vi "Exit CMD.vi"(11 "Close Panel on Exit?":bool) -> (3 "Exit CMD":string)   [LabVIEW 2017]
doc: "函数名称： \n函数功能：JKI状态机 退出命令 （退出前输出输出数据） \n入口参数：\n出口参数：\n创建时间：2018-8-14 编辑者 ：翁赟\n---------------------------------------------------------------------\n修改时间：\n修改备注： 注意状态机里 命令是否符合"
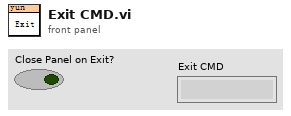
[diagram p1: front panel]
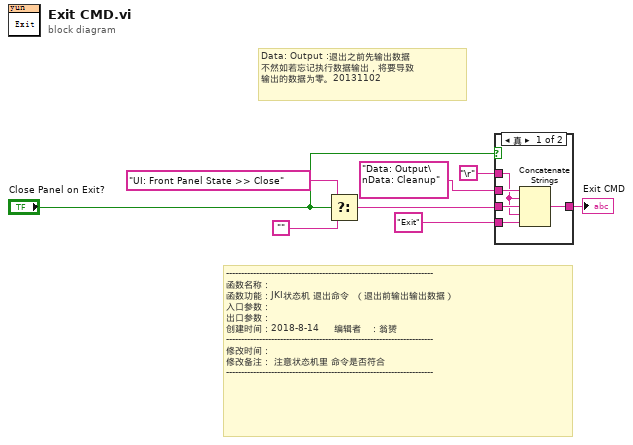
[diagram p0: block diagram]
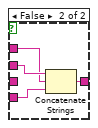
[diagram p2: hidden frame]
diagram:
  # "---------------------------------------------------------------------\n函数名称： \n函数功能：JKI状态机 退出命令  （退出前输出输出数据） \n入口参数：\n出口参数：\n创建时间：2018-8-14     编辑者   ：翁赟\n---------------------------------------------------------------------\n修改时间：\n修改备注： 注意状态机里 命令是否符合\n---------------------------------------------------------------------"
  # "Data: Output :退出之前先输出数据\n不然如若忘记执行数据输出，将要导致\n输出的数据为零。20131102"
  n1 = Select(t="UI: Front Panel State >> Close", s="Close Panel on Exit?", f="") -> (s? t:f=w8:string)
  n2 = case shown="真" "Close Panel on Exit?" {
    tunnel: w8 -> [w12 _]
    tunnel: "Data: Output\nData: Cleanup" -> [w13 w17]
    tunnel: "\r" -> [w11 w16]
    tunnel: "Exit" -> [w10 w15]
    tunnel: [w9 w14] -> w1
    frame True {
      n3 = Concatenate Strings(w13, w11, w12, w11, w10) -> (w9:string)
    }
    frame False {
      n4 = Concatenate Strings(w17, w16, w15) -> (w14:string)
    }
  }
  "Exit CMD" <- w1
